vi "Start New Edit.vi"(8 "error in (no error)":errorcluster, 10 "New Search":refnum<class "Search.lvclass">, 11 "BetterSearch in":refnum<class "BetterSearch.lvclass">) -> (0 "error out":errorcluster, 3 "BetterSearch out":refnum<class "BetterSearch.lvclass">)   [LabVIEW 2016, in "Better Search.lvlib" / "BetterSearch.lvclass"]
uses:
  BetterSearch.lvclass
  Search/Search.lvclass
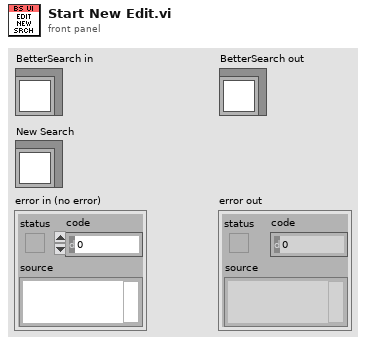
[diagram p1: front panel]
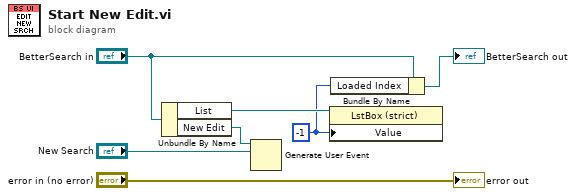
[diagram p0: block diagram]
diagram:
  w2 = -1 ("Value")
  n1 = Unbundle By Name("BetterSearch in") -> ("List"=w4:refnum<vi>, "New Edit"=w6:refnum<user-event>)
  n2 = Generate User Event(user event=w6, event data cluster="New Search") -> ()  [unwired: 2 in, 2 out]
  n3 = property class="LstBox (strict)"(reference=w4, "Value"=w2) -> ()  [unwired: 1 in, 2 out]
  n4 = Bundle By Name(cluster="BetterSearch in", "Loaded Index"=w2) -> (→"BetterSearch out":refnum<class "BetterSearch.lvclass">)
  "error out" <- "error in (no error)"
